vi "for loop.vi"() -> ()   [LabVIEW 2020]
uses:
  Control 1.ctl
panel:
  in  "Cluster":T1
  out "Waveform Chart":i32(graph)
  out "Sum":i32
  in  "Numeric":u32
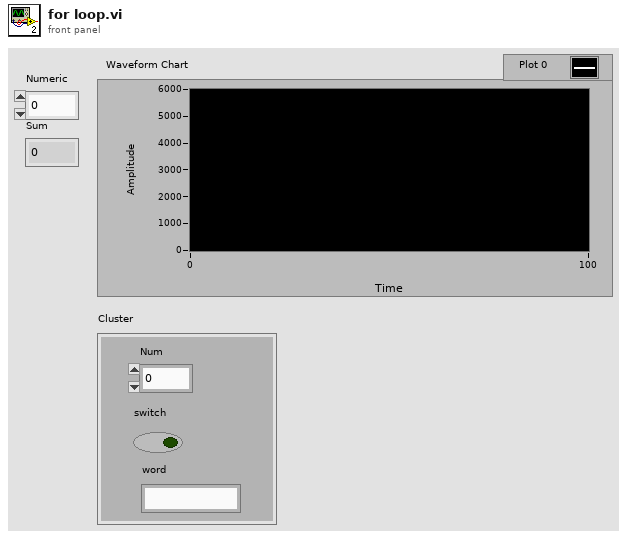
[diagram p1: front panel]
types:
  T1 = typedef "Control 1.ctl" = cluster{"Num":dbl, "switch":bool, "word":string}
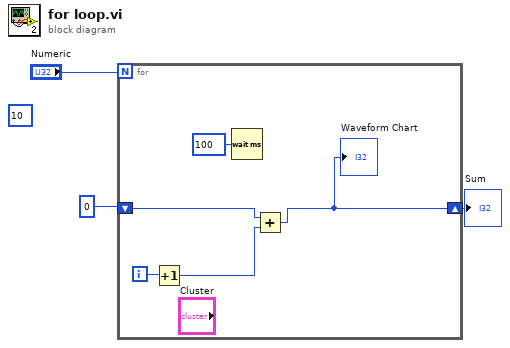
[diagram p0: block diagram]
diagram:
  (unwired) u32 10 ("Numeric")
  n1 = for {
    N: "Numeric" -> [_]
    shift-right: [w5] -> w2
    shift-left: 0 -> [w7]
    i -> [w8]
    n2 = Increment(x=w8) -> (x+1=w6:i32)
    n3 = Wait (ms)(milliseconds to wait=u32 100) -> ()  [unwired: 1 out]
    n4 = Add(x=w7, y=w6) -> (x+y=w5:i32)
    "Waveform Chart" <- w5
  }
  "Sum" <- w2
